vi "Build Array with Memory.vi"(5 "reset":bool, 7 "max array length":i32=-1, 10 "new array":dbl[](array[numeric])) -> (2 "appended array":dbl[](array[numeric]))   [LabVIEW 2019]
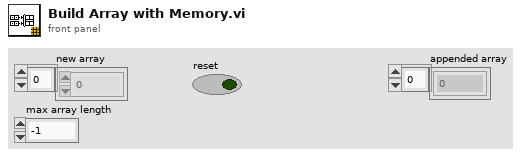
[diagram p1: front panel]
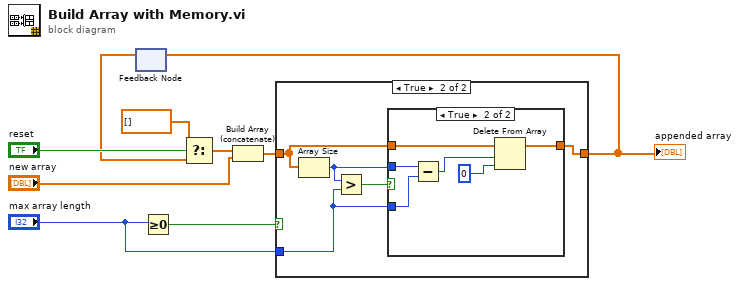
[diagram p0: block diagram]
diagram:
  n1 = feedback #1() -> (w2:dbl[])  [unwired: 1 in]
  n2 = Greater Or Equal To 0?(x="max array length") -> (x >= 0?=w9:bool)
  n3 = Select(t=dbl[] [], s="reset", f=w2) -> (s? t:f=w5:dbl[])
  n4 = Build Array (concatenate)(w5, "new array") -> (w4:dbl[])
  n5 = case shown="True" w9 {
    tunnel: [w10 w15] -> w3
    tunnel: w4 -> [w10 w14]
    tunnel: "max array length" -> [_ w12]
    frame False {
    }
    frame True {
      n6 = Array Size(array=w14) -> (size(s)=w11:i32)
      n7 = Greater?(x=w11, y=w12) -> (0:w13:bool)
      n8 = case shown="True" w13 {
        tunnel: [w16 w22] -> w15
        tunnel: w14 -> [w16 w20]
        tunnel: w12 -> [_ w18]
        tunnel: w11 -> [_ w19]
        frame False {
        }
        frame True {
          n9 = Subtract(x=w19, y=w18) -> (x-y=w17:i32)
          n10 = Delete From Array(array=w20, length=w17, index=0) -> (array with subset deleted=w22:dbl[])  [unwired: 1 out]
        }
      }
    }
  }
  "appended array" <- w3
  n11 = feedback-in #1(w3) -> ()
